vi "EditorThumbnail mouseDown.vi"(7 "coordsHorizontal":i32, 8 "error in (no error)":errorcluster, 11 "EditorThumbnail in":refnum<class "EditorThumbnail.lvclass">) -> (0 "error out":errorcluster, 3 "EditorThumbnail out":refnum<class "EditorThumbnail.lvclass">, 5 "index":u32)   [LabVIEW 2018, in "EditorThumbnail.lvclass"]
uses:
  EditorThumbnail.lvclass
  EditorThumbnail.lvclass/EditorThumbnail.ctl
  <vilib>/Utility/miscctls.llb/LVPositionTypeDef.ctl
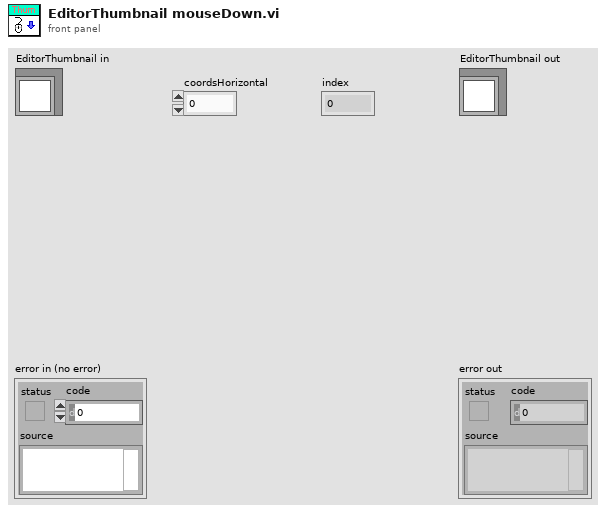
[diagram p1: front panel]
types:
  T1 = cluster{"index":u32, "data":cluster{"xdata":dbl[], "ydata":sgl[]}[], "peak":dbl[], "picture":picture}
  T2 = typedef "LVPositionTypeDef.ctl" = cluster{"Left":i32, "Top":i32}
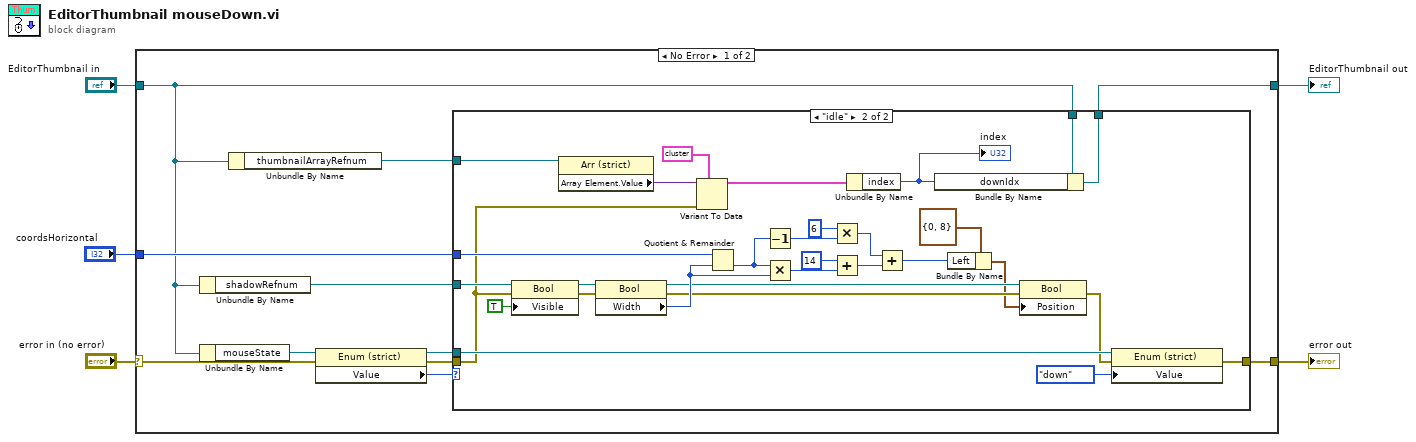
[diagram p0: block diagram]
diagram:
  n1 = case shown="No Error" "error in (no error)" {
    selector: "error in (no error)" -> [w13 w50]
    tunnel: [w11 w50] -> w4
    tunnel: [w8 w49] -> w2
    tunnel: "EditorThumbnail in" -> [w6 w49]
    tunnel: "coordsHorizontal" -> [w9 _]
    frame No Error {
      n2 = Unbundle By Name(w6) -> ("shadowRefnum"=w10:refnum<vi>)
      n3 = Unbundle By Name(w6) -> ("mouseState"=w16:refnum<vi>)
      n4 = Unbundle By Name(w6) -> ("thumbnailArrayRefnum"=w7:refnum<vi>)
      n5 = property class="Enum (strict)"(reference=w16, error in=w13) -> (reference out=w14:refnum<vi>, error out=w12:errorcluster, "Value"=w15:enum16{"idle", "down", "move", "up"})
      n6 = case shown="\"idle\"" w15 {
        tunnel: w14 -> [_ w48]
        tunnel: w12 -> [w18 w19]
        tunnel: [w18 w46] -> w11
        tunnel: w10 -> [_ w43]
        tunnel: w9 -> [_ w33]
        tunnel: w6 -> [w17 w27]
        tunnel: [w17 w26] -> w8
        tunnel: w7 -> [_ w25]
        frame Default {
        }
        frame "idle" {
          n7 = property class="Bool"(reference=w43, error in=w19, "Visible"=TRUE) -> (reference out=w45:refnum<vi>, error out=w44:errorcluster)
          n8 = property class="Arr (strict)"(reference=w25) -> ("Array Element.Value"=w24:variant)  [unwired: 1 in, 2 out]
          n9 = property class="Bool"(reference=w45, error in=w44) -> (reference out=w32:refnum<vi>, error out=w31:errorcluster, "Width"=w34:u32)
          n10 = Variant To Data(error in=w19, type=T1 {"index"=0, "data"=[], "peak"=[], "picture"=bytes[0]} ("ThumbnailFormat"), Variant=w24) -> (data=w23:T1)  [unwired: 1 out]
          n11 = Quotient & Remainder(x=w33, y=w34) -> (floor(x/y)=w41:u32)  [unwired: 1 out]
          n12 = Decrement(x=w41) -> (x-1=w36:u32)
          n13 = Multiply(x=w41, y=w34) -> (x*y=w40:u32)
          n14 = Multiply(x=u32 6 ("y"), y=w36) -> (x*y=w35:u32)
          n15 = Add(x=u32 14, y=w40) -> (x+y=w38:u32)
          n16 = Unbundle By Name(w23) -> ("index"=w22:u32)
          "index" <- w22
          n17 = Add(x=w35, y=w38) -> (x+y=w20:u32)
          n18 = Bundle By Name(cluster=w27, "downIdx"=w22) -> (w26:refnum<class "EditorThumbnail.lvclass">)
          n19 = Bundle By Name(cluster=T2 {"Left"=0, "Top"=8} ("Position"), "Left"=w20) -> (w29:T2)
          n20 = property class="Bool"(reference=w32, error in=w31, "Position"=w29) -> (error out=w28:errorcluster)  [unwired: 1 out]
          n21 = property class="Enum (strict)"(reference=w48, error in=w28, "Value"=enum16{"idle", "down", "move", "up"}."down") -> (error out=w46:errorcluster)  [unwired: 1 out]
        }
      }
    }
    frame Error {
    }
  }
  "error out" <- w4
  "EditorThumbnail out" <- w2
